vi "超标留样全局.vi"() -> ()   [LabVIEW 2022 SP3, in "超标留样集成.lvlib" / "科盛超标留样.lvlib"]
panel:
  out "查询采样记录":T1(array[cluster])
  out "查询瓶记录":T2
  out "通讯":bool
  out "留样等待时间":dbl
  out "供样等待时间":dbl
  out "采样等待时间":dbl
  out "流程中":bool
  out "超标留样信号":bool
  out "开关量3状态":T3
  out "开关量2状态":T4
  out "开关量1状态":T5
  out "查询系统状态":T6
  out "留样完成":bool
  out "采样完成":bool
  out "供样完成":bool
  in  "VISA resource name":refnum<visa-resource-name>="COM2" caption="VISA资源名称"
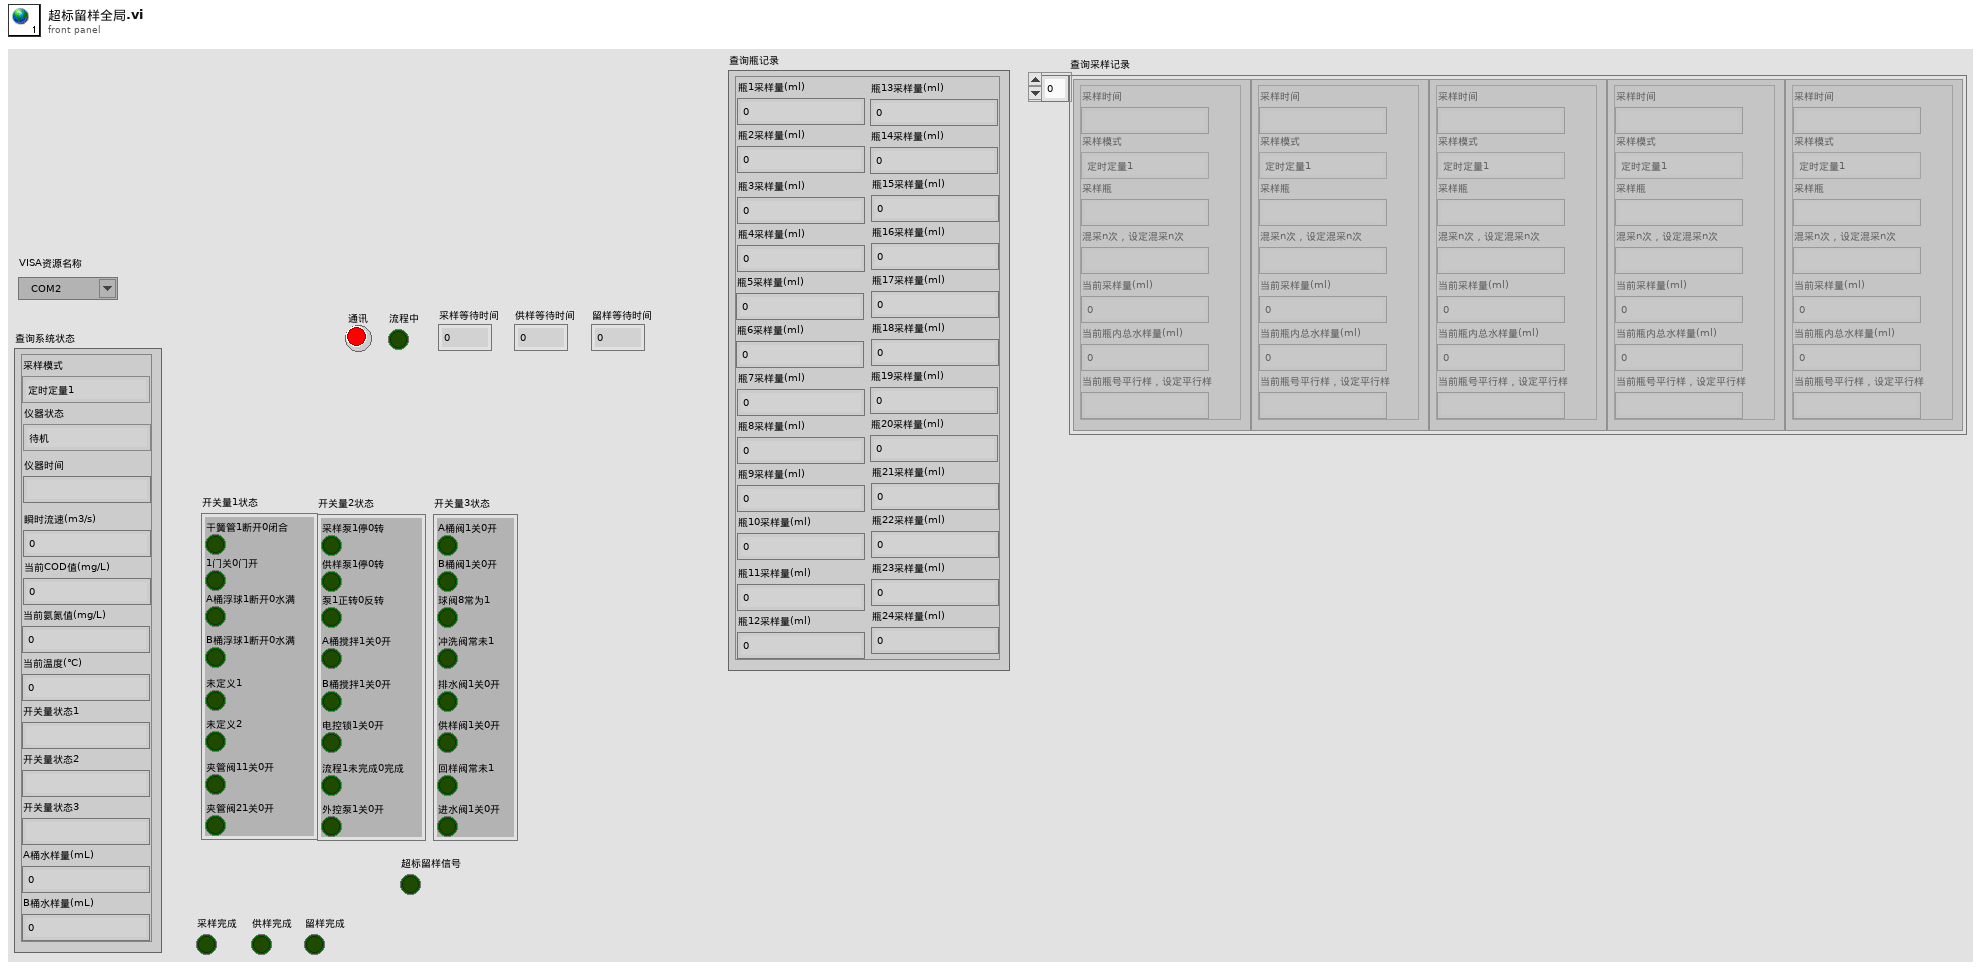
[diagram p1: front panel]
types:
  T1 = cluster{"采样时间":string, "采样模式":enum16{"定时定量1", "定时定量2", "定流定量", "定时比例", "同步留样", "超标留样", "触发采样", "定时采样1", "定流供样", "定时采样2", "远程取样", "手动取样", "流量跟踪"}, "采样瓶":string, "混采n次，设定混采n次":string, "当前采样量(ml)":dbl, "当前瓶内总水样量(ml)":dbl, "当前瓶号平行样，设定平行样":string}[]
  T2 = cluster{"瓶1采样量(ml)":dbl, "瓶2采样量(ml)":dbl, "瓶3采样量(ml)":dbl, "瓶4采样量(ml)":dbl, "瓶5采样量(ml)":dbl, "瓶6采样量(ml)":dbl, "瓶7采样量(ml)":dbl, "瓶8采样量(ml)":dbl, "瓶9采样量(ml)":dbl, "瓶10采样量(ml)":dbl, "瓶11采样量(ml)":dbl, "瓶12采样量(ml)":dbl, "瓶13采样量(ml)":dbl, "瓶14采样量(ml)":dbl, "瓶15采样量(ml)":dbl, "瓶16采样量(ml)":dbl, "瓶17采样量(ml)":dbl, "瓶18采样量(ml)":dbl, "瓶19采样量(ml)":dbl, "瓶20采样量(ml)":dbl, "瓶21采样量(ml)":dbl, "瓶22采样量(ml)":dbl, "瓶23采样量(ml)":dbl, "瓶24采样量(ml)":dbl}
  T3 = cluster{"A桶阀1关0开":bool, "B桶阀1关0开":bool, "球阀8常为1":bool, "冲洗阀常未1":bool, "排水阀1关0开":bool, "供样阀1关0开":bool, "回样阀常未1":bool, "进水阀1关0开":bool}
  T4 = cluster{"采样泵1停0转":bool, "供样泵1停0转":bool, "泵1正转0反转":bool, "A桶搅拌1关0开":bool, "B桶搅拌1关0开":bool, "电控锁1关0开":bool, "流程1未完成0完成":bool, "外控泵1关0开":bool}
  T5 = cluster{"干簧管1断开0闭合":bool, "1门关0门开":bool, "A桶浮球1断开0水满":bool, "B桶浮球1断开0水满":bool, "未定义1":bool, "未定义2":bool, "夹管阀11关0开":bool, "夹管阀21关0开":bool}
  T6 = cluster{"采样模式":enum16{"定时定量1", "定时定量2", "定流定量", "定时比例", "同步留样", "超标留样", "触发采样", "定时采样1", "定流供样", "定时采样2", "远程取样", "手动取样", "流量跟踪"}, "仪器状态":enum16{"待机", "运行中"}, "仪器时间":string, "瞬时流速(m3/s)":dbl, "当前COD值(mg/L)":dbl, "当前氨氮值(mg/L)":dbl, "当前温度(℃)":dbl, "开关量状态1":string, "开关量状态2":string, "开关量状态3":string, "A桶水样量(mL)":dbl, "B桶水样量(mL)":dbl}
diagram:
